vi "Query Status Register.vi"(8 "error in":errorcluster, 11 "69X_79X in":refnum<class "7976A.lvclass">) -> (0 "error out":errorcluster, 3 "69X_79X out":refnum<class "7976A.lvclass">)   [LabVIEW 2019, in "7976A.lvlib" / "7976A.lvclass"]
doc: "Child classes must override this VI:\n\nThis VI is the device specific query of the supply's status registers. \nThe return values are: \n\nThe implementation must read status registers and push the status register values to private data for:\nOCP Flag, OVP Flag, Interlock Flag, Output Flag into the private data arrays of the power supply class."
uses:
  Library/7976A.lvclass
  C:/Users/Public/Documents/Development/builds/Instruments/PowerSupply.lvlibp/Library/PowerSupply.lvclass
  builds/Instruments/PowerSupply.lvlibp/Custom Controls/Status_Flags.ctl
  Library/7976A.lvclass/7976A.ctl
  builds/Instruments/PowerSupply.lvlibp/Accessors/Write Status Flags.vi
  builds/Instruments/PowerSupply.lvlibp/Library/PowerSupply.lvclass
  builds/Engine/Engine.lvlibp/Project/Engine.lvclass
  <instrlib>/Agilent N7976A/Agilent N7976A.lvlib
  C:/Users/Public/Documents/Development/builds/Engine/Engine.lvlibp/Project/Engine.lvclass
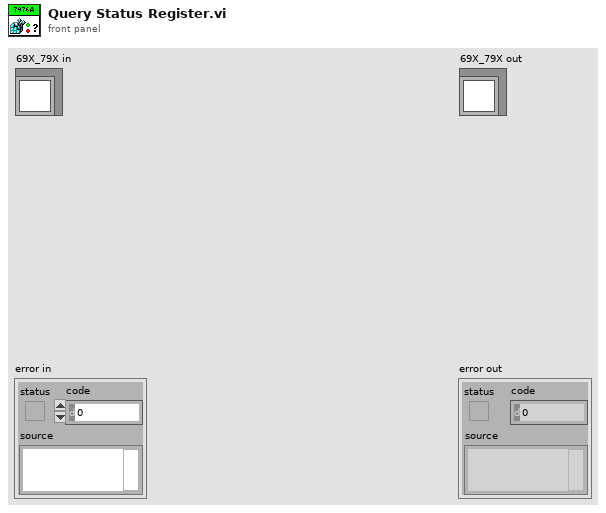
[diagram p1: front panel]
types:
  T1 = typedef "PowerSupply.lvlibp/PowerSupply.lvclass/Status_Flags.ctl" = cluster{"Interlock":bool, "OVP":bool, "OCP":bool, "Output":bool}
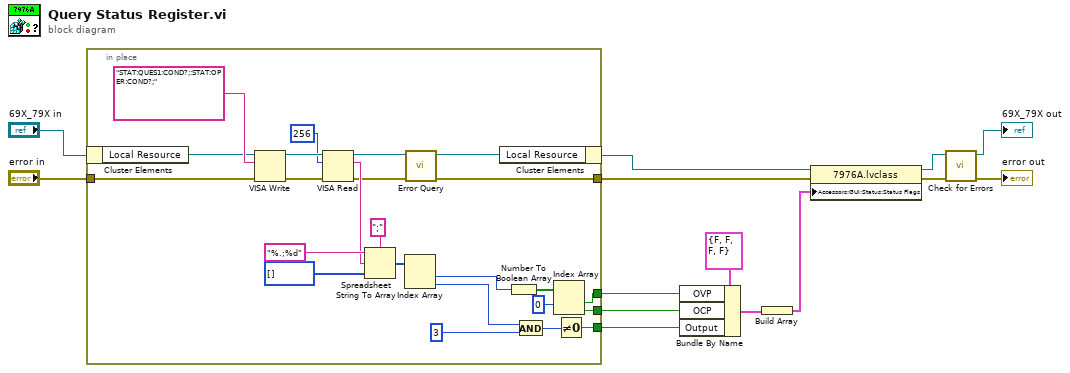
[diagram p0: block diagram]
diagram:
  n1 = in-place {
    in-place-border: "error in" -> [w33]
    in-place-border: [w16] -> w8
    in-place-border: [w23] -> w12
    in-place-border: [w20] -> w10
    in-place-border: [w19] -> w11
    n2 = in-place-cluster #1("69X_79X in") -> ("Local Resource"=w35:refnum<visa-resource-name>)
    n3 = VISA Write(VISA resource name=w35, write buffer="STAT:QUES1:COND?;:STAT:OPER:COND?;", error in (no error)=w33) -> (VISA resource name out=w38:refnum<visa-resource-name>, error out=w37:errorcluster)  [unwired: 1 out]
    n4 = VISA Read(VISA resource name=w38, byte count=u32 256, error in (no error)=w37) -> (VISA resource name out=w18:refnum<visa-resource-name>, read buffer=w29:string, error out=w17:errorcluster)  [unwired: 1 out]
    n5 = Spreadsheet String To Array(delimiter (Tab)=";", format string="%.;%d", spreadsheet string=w29, array type (2D Dbl)=u32[] []) -> (array=w28:u32[])
    n6 = Index Array(array=w28) -> (element #1=w27:u32, element #2=w26:u32)  [unwired: 2 in]
    n7 = call <instrlib>:"Error Query.vi"("error in (no error)"=w17, "VISA resource name"=w18) -> ("error out"=w16:errorcluster, "VISA resource name out"=w15:refnum<visa-resource-name>)  [unwired: 6 in, 2 out]
    n8 = in-place-cluster #1("Local Resource"=w15) -> (w7:refnum<class "7976A.lvclass">)
    n9 = Number To Boolean Array(number=w27) -> (Boolean array=w22:bool[])
    n10 = And(x=w26, y=u32 3 ("x")) -> (x .and. y?=w24:u32)
    n11 = Index Array(array=w22, index #1=0 ("index")) -> (element #1=w20:bool, element #2=w19:bool)  [unwired: 1 in]
    n12 = Not Equal To 0?(x=w24) -> (x != 0?=w23:bool)
  }
  n13 = Bundle By Name(cluster=T1 {"Interlock"=FALSE, "OVP"=FALSE, "OCP"=FALSE, "Output"=FALSE} ("Status"), "OVP"=w10, "OCP"=w11, "Output"=w12) -> (w13:T1)
  n14 = Build Array(w13) -> (w14:T1[])
  n15 = property class="7976A.lvclass"(reference=w7, error in=w8, "Accessors:GUI:Status:Status Flags"=w14) -> (reference out=w2:refnum<class "7976A.lvclass">, error out=w1:errorcluster)
  n16 = call "Check for Errors.vi"("error in"=w1, "Engine in"=w2) -> ("error out"=→"error out":errorcluster, "Engine out"=→"69X_79X out":refnum<class "7976A.lvclass">)  [unwired: 8 in]
